vi "DHE_ReadExpTPs.vi"(8 "error in (no error)":errorcluster, 11 "fd":i32) -> (0 "error out":errorcluster)   [LabVIEW 2016]
uses:
  private/vis/DHE_TP_action.ctl
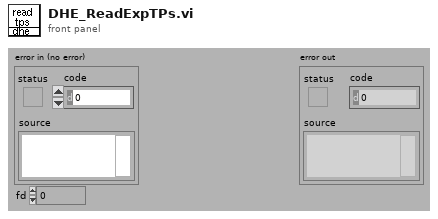
[diagram p1: front panel]
types:
  T1 = typedef "DHE_TP_action.ctl" = enum16{"READ FROM FILE", "GET ALL", "FIND BY NAME", "FIND BY TYPE", "SET VALUE", "CLEAN", "CHANGE", "GET EXPUPDATE"}
  T2 = typedef "DHE_TP.ctl" = cluster{"name":string, "type":string, "R_algor":string[], "board":string, "memory":string, "address":i32, "value":string, "Limits":T3, "unit":string, "params":string, "permissions":string, "W_algor":string[], "description":string, "err_count":i32, "max_err":i32, "read":bool, "lowrej":dbl, "hirej":dbl, "expupd":bool}
  T3 = typedef "DHE_TPLimits.ctl" = cluster{"upper":dbl, "Lower":dbl, "InRange":bool, "nominal":dbl}
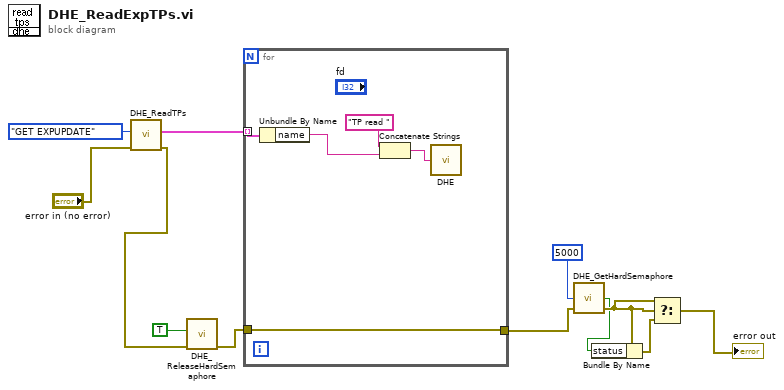
[diagram p0: block diagram]
diagram:
  n1 = call "DHE_ReadTPs.vi"("error in (no error)"="error in (no error)", "action"=DHE_TP_action."GET EXPUPDATE") -> ("error out"=w7:errorcluster, "TPs"=w6:T2[])  [unwired: 5 in, 3 out]
  n2 = call "DHE_ReleaseHardSemaphore.vi"("error in (no error)"=w7, "release?"=TRUE) -> ("error out"=w11:errorcluster)  [unwired: 9 out]
  n3 = for {
    tunnel: w11 -> [w17]
    tunnel: [w17] -> w10
    tunnel: w6 -> [w16] mode=indexing
    n4 = Unbundle By Name(w16) -> ("name"=w13:string)
    n5 = Concatenate Strings("TP read " ("string"), w13) -> (w14:string)
    n6 = call "DHE.vi"("Cmd"=w14) -> ()  [unwired: 2 in, 13 out]
  }
  n7 = call "DHE_GetHardSemaphore.vi"("timeout"=5000, "error in (no error)"=w10) -> ("timed out"=w2:bool, "error out"=w3:errorcluster)  [unwired: 6 out]
  n8 = Bundle By Name(cluster=w3, "status"=w2) -> (w1:errorcluster)
  n9 = Select(t=w3, s=w3, f=w1) -> (s? t:f=→"error out":errorcluster)
